vi "Create IO Channels.vi"(6 "AI Buffer Size (s)":i32=10, 8 "AI Block Size":i32=5000, 9 "OSC Configuration":T3(array[cluster])=[[{"Signal Type"=enum."Sine Wave", "DC"=0.0, "Amplitude"=0.01, "frequency"=2.0, "Phase"=0.0}, {"Signal Type"=enum."Sine Wave", "DC"=0.001, "Amplitude"=0.005, "frequency"=2.0, "Phase"=0.0}]] {"frequency" step=0.001 format="%.3p"; "Amplitude" format="%0.2p"; "DC" min=-0.99 max=0.99 format="%.2p"}, 10 "AO Configuration":T1(array[cluster])=[{"Output physical channels"="PXI1Slot2/ao0", "AO. Max"=0.1, "AO.Min"=-0.1}, {"Output physical channels"="", "AO. Max"=0.1, "AO.Min"=-0.1}], 11 "AI Configuration":T2(array[cluster])=[{"AI.Coupling"=10050, "AI.Max"=10.0, "AI.Min"=-10.0, "Input physical channels"="PXI1Slot2/ai0:1"}, {"AI.Coupling"=10050, "AI.Max"=10.0, "AI.Min"=-10.0, "Input physical channels"="PXI1Slot3/ai0:3"}, {"AI.Coupling"=10050, "AI.Max"=10.0, "AI.Min"=-10.0, "Input physical channels"=""}] {"AI.Coupling" items=["AC"=10045, "DC"=10050, "GND"=10066]}) -> (0 "Sampling information":cluster{"Fs":dbl, "#s":dbl}[](array[cluster])=[{"Fs"=10000.0, "#s"=5000.0}, {"Fs"=10000.0, "#s"=5000.0}], 1 "AI Rate":dbl=10000.0 format="%.2f", 2 "AO Task":refnum<k21>[](array[refnum]), 3 "AI task":refnum<k21>[](array[refnum]), 4 "phase log":dbl[](array[numeric])=[0.99999999999938, 0.99999999999938], 5 "appended array":errorcluster[][](array[cluster]))   [LabVIEW 2013]
uses:
  <vilib>/DAQmx/create/channels.llb/DAQmx Create Channel (AI-Voltage-Basic).vi
  <vilib>/DAQmx/configure/timing.llb/DAQmx Timing (Sample Clock).vi
  Lock-in Globals Multiple Inputs and Outputs.vi
  <vilib>/DAQmx/create/channels.llb/DAQmx Create Channel (AO-Voltage-Basic).vi
  <vilib>/DAQmx/configure/trigger.llb/DAQmx Start Trigger (Digital Edge).vi
  <vilib>/DAQmx/write.llb/DAQmx Write (Analog 1D Wfm NChan NSamp).vi
  <resource>/objmgr/daqmx.rc
  <vilib>/measure/NI_MABase.lvlib
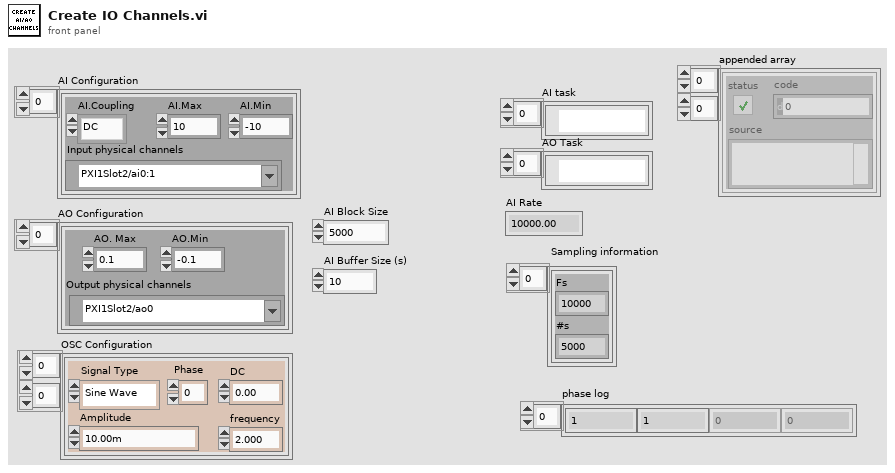
[diagram p1: front panel]
types:
  T1 = cluster{"Output physical channels":tag, "AO. Max":dbl, "AO.Min":dbl}[]
  T2 = cluster{"AI.Coupling":i32, "AI.Max":dbl, "AI.Min":dbl, "Input physical channels":tag}[]
  T3 = cluster{"Signal Type":enum16{"Sine Wave", "Triangle Wave", "Square Wave", "Sawtooth Wave"}, "DC":dbl, "Amplitude":dbl, "frequency":dbl, "Phase":dbl}[][]
  T4 = cluster{"AI.Coupling":i32, "AI.Max":dbl, "AI.Min":dbl, "Input physical channels":tag}
  T5 = cluster{"Signal Type":enum16{"Sine Wave", "Triangle Wave", "Square Wave", "Sawtooth Wave"}, "DC":dbl, "Amplitude":dbl, "frequency":dbl, "Phase":dbl}
  T6 = enum16{"Sine Wave", "Triangle Wave", "Square Wave", "Sawtooth Wave"}
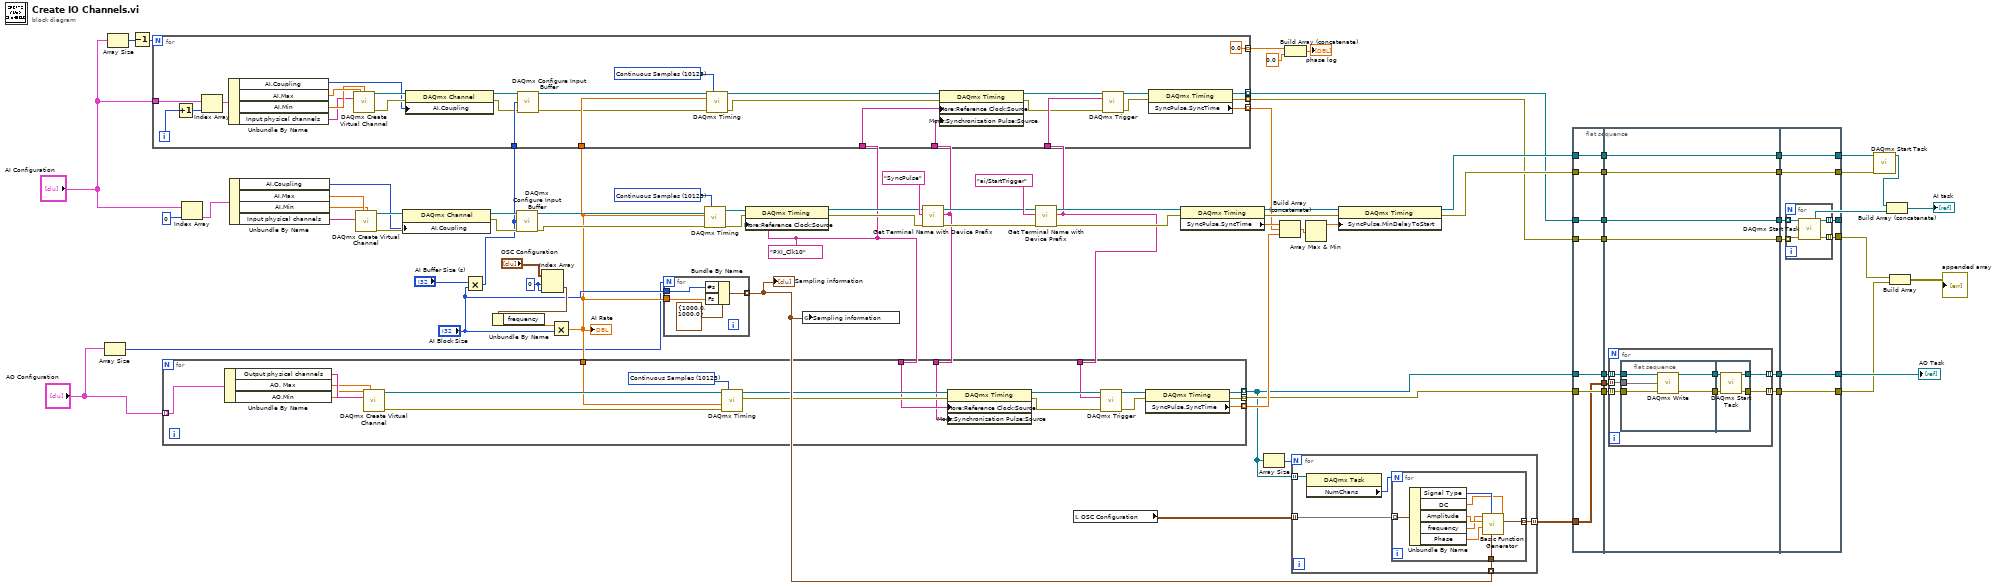
[diagram p0: block diagram]
diagram:
  w19 = 0 ("index (row)")
  w17 = tag "PXI_Clk10" ("RefClk.Src")
  w66 = 10123 items=["Finite Samples"=10178, "Continuous Samples"=10123] ("sample mode")
  n1 = Array Size(array="AO Configuration") -> (size(s)=w1:i32)
  n2 = Array Size(array="AI Configuration") -> (size(s)=w22:i32)
  n3 = Decrement(x=w22) -> (x-1=w21:i32)
  n4 = Index Array(array="AI Configuration", index=0) -> (element=w67:T4)
  n5 = Unbundle By Name(w67) -> ("AI.Coupling"=w39:i32, "AI.Max"=w46:dbl, "AI.Min"=w45:dbl, "Input physical channels"=w47:tag)
  n6 = call-poly <vilib>:"DAQmx Create Virtual Channel.vi"("maximum value"=w46, "minimum value"=w45, "physical channels"=w47) -> ("task out"=w41:refnum<k21>, "error out"=w40:errorcluster)  [unwired: 11 in]
  n7 = property class="DAQmx Channel"(reference=w41, error in=w40, "AI.Coupling"=w39) -> (reference out=w38:refnum<k21>, error out=w37:errorcluster)
  n8 = Multiply(x="AI Buffer Size (s)", y="AI Block Size") -> (x*y=w20:i32)
  n9 = call <vilib>:"DAQmx Configure Input Buffer.vi"("task/channels in"=w38, "buffer size (in samples per channel)"=w20, "error in"=w37) -> ("task out"=w36:refnum<k21>, "error out"=w35:errorcluster)  [unwired: 11 in]
  n10 = Index Array(array="OSC Configuration", index (row)=w19, index (col)=w19) -> (element=w30:T5)
  n11 = Unbundle By Name(w30) -> ("frequency"=w29:dbl)
  n12 = Multiply(x=w29, y="AI Block Size") -> (x*y=w18:dbl)
  "AI Rate" <- w18
  n13 = for {
    N: w1 -> [_]
    tunnel: w18 -> [w85]
    tunnel: "AI Block Size" -> [w84]
    tunnel: [w82] -> w8 mode=indexing
    n14 = Bundle By Name(cluster=cluster{"Fs":dbl, "#s":dbl} {"Fs"=1000.0, "#s"=1000.0} ("sampling info"), "#s"=w84, "Fs"=w85) -> (w82:cluster{"Fs":dbl, "#s":dbl})
  }
  "Sampling information" <- w8
  n15 = call-poly <vilib>:"DAQmx Timing.vi"("task/channels in"=w36, "sample mode"=w66, "rate"=w18, "error in"=w35) -> ("task out"=w65:refnum<k21>, "error out"=w64:errorcluster)  [unwired: 10 in]
  n16 = property class="DAQmx Timing"(reference=w65, error in=w64, "More:Reference Clock:Source"=w17) -> (reference out=w43:refnum<k21>, error out=w42:errorcluster)
  n17 = global write "Lock-in Globals Multiple Inputs and Outputs.vi" "Sampling information"(w8) -> ()
  n18 = call <userlib>:"Get Terminal Name with Device Prefix.vi"("error in (no error)"=w42, "Local Terminal Name"="SyncPulse", "task/channels in"=w43) -> ("error out"=w59:errorcluster, "Terminal Name with Device Prefix"=w16:tag, "task out"=w60:refnum<k21>)  [unwired: 6 in]
  n19 = call <userlib>:"Get Terminal Name with Device Prefix.vi"("error in (no error)"=w59, "Local Terminal Name"="ai/StartTrigger", "task/channels in"=w60) -> ("error out"=w57:errorcluster, "Terminal Name with Device Prefix"=w26:tag, "task out"=w58:refnum<k21>)  [unwired: 6 in]
  n20 = for {
    N: w21 -> [_]
    tunnel: "AI Configuration" -> [w113]
    tunnel: w20 -> [w115]
    tunnel: w18 -> [w114]
    tunnel: w17 -> [w112]
    tunnel: w16 -> [w111]
    tunnel: w26 -> [w110]
    tunnel: [w109] -> w25 mode=indexing
    tunnel: [w108] -> w23 mode=indexing
    tunnel: [w107] -> w24 mode=indexing
    tunnel: [0.0] -> w12 mode=indexing
    i -> [w88]
    w97 = 10123 items=["Finite Samples"=10178, "Continuous Samples"=10123, "Hardware Timed Single Point"=12522] ("sample mode")
    n21 = Increment(x=w88) -> (x+1=w87:i32)
    n22 = Index Array(array=w113, index=w87) -> (element=w96:T4)
    n23 = Unbundle By Name(w96) -> ("AI.Coupling"=w101:i32, "AI.Max"=w106:dbl, "AI.Min"=w105:dbl, "Input physical channels"=w104:tag)
    n24 = call-poly <vilib>:"DAQmx Create Virtual Channel.vi"("maximum value"=w106, "minimum value"=w105, "physical channels"=w104) -> ("task out"=w102:refnum<k21>, "error out"=w103:errorcluster)  [unwired: 11 in]
    n25 = property class="DAQmx Channel"(reference=w102, error in=w103, "AI.Coupling"=w101) -> (reference out=w100:refnum<k21>, error out=w99:errorcluster)
    n26 = call <vilib>:"DAQmx Configure Input Buffer.vi"("task/channels in"=w100, "buffer size (in samples per channel)"=w115, "error in"=w99) -> ("task out"=w98:refnum<k21>, "error out"=w91:errorcluster)  [unwired: 11 in]
    n27 = call-poly <vilib>:"DAQmx Timing.vi"("task/channels in"=w98, "sample mode"=w97, "rate"=w114, "error in"=w91) -> ("task out"=w95:refnum<k21>, "error out"=w90:errorcluster)  [unwired: 10 in]
    n28 = property class="DAQmx Timing"(reference=w95, error in=w90, "More:Reference Clock:Source"=w112, "More:Synchronization Pulse:Source"=w111) -> (reference out=w94:refnum<k21>, error out=w89:errorcluster)
    n29 = call-poly <vilib>:"DAQmx Trigger.vi"("task/channels in"=w94, "source"=w110, "error in"=w89) -> ("task out"=w93:refnum<k21>, "error out"=w92:errorcluster)  [unwired: 11 in]
    n30 = property class="DAQmx Timing"(reference=w93, error in=w92) -> (reference out=w107:refnum<k21>, error out=w108:errorcluster, "SyncPulse.SyncTime"=w109:dbl)
  }
  n31 = for {
    tunnel: [w128] -> w51 mode=indexing
    tunnel: [w127] -> w48 mode=indexing
    tunnel: [w121] -> w9 mode=indexing
    tunnel: w26 -> [w120]
    tunnel: "AO Configuration" -> [w116] mode=indexing
    tunnel: w18 -> [w119]
    tunnel: w17 -> [w118]
    tunnel: w16 -> [w117]
    w135 = 10123 items=["Finite Samples"=10178, "Continuous Samples"=10123] ("sample mode")
    n32 = Unbundle By Name(w116) -> ("Output physical channels"=w124:tag, "AO. Max"=w123:dbl, "AO.Min"=w122:dbl)
    n33 = call-poly <vilib>:"DAQmx Create Virtual Channel.vi"("maximum value"=w123, "minimum value"=w122, "physical channels"=w124) -> ("task out"=w126:refnum<k21>, "error out"=w125:errorcluster)  [unwired: 11 in]
    n34 = call-poly <vilib>:"DAQmx Timing.vi"("task/channels in"=w126, "sample mode"=w135, "rate"=w119, "error in"=w125) -> ("task out"=w134:refnum<k21>, "error out"=w133:errorcluster)  [unwired: 10 in]
    n35 = property class="DAQmx Timing"(reference=w134, error in=w133, "More:Reference Clock:Source"=w118, "More:Synchronization Pulse:Source"=w117) -> (reference out=w132:refnum<k21>, error out=w131:errorcluster)
    n36 = call-poly <vilib>:"DAQmx Trigger.vi"("task/channels in"=w132, "source"=w120, "error in"=w131) -> ("task out"=w129:refnum<k21>, "error out"=w130:errorcluster)  [unwired: 11 in]
    n37 = property class="DAQmx Timing"(reference=w129, error in=w130) -> (reference out=w121:refnum<k21>, error out=w127:errorcluster, "SyncPulse.SyncTime"=w128:dbl)
  }
  n38 = local read "OSC Configuration"() -> (w27:T3)
  n39 = property class="DAQmx Timing"(reference=w58, error in=w57) -> (reference out=w54:refnum<k21>, error out=w55:errorcluster, "SyncPulse.SyncTime"=w56:dbl)
  n40 = Array Size(array=w9) -> (size(s)=w10:i32)
  n41 = Build Array (concatenate)(w56, w25, w51) -> (w53:dbl[])
  n42 = Build Array (concatenate)(w12, 0.0) -> (→"phase log":dbl[])
  n43 = for {
    N: w10 -> [_]
    tunnel: w27 -> [w140] mode=indexing
    tunnel: [w139] -> w15 mode=indexing
    tunnel: w9 -> [w137] mode=indexing
    tunnel: w8 -> [w136] mode=indexing
    n44 = property class="DAQmx Task"(reference=w137) -> ("NumChans"=w138:u32)  [unwired: 1 in, 2 out]
    n45 = for {
      N: w138 -> [_]
      tunnel: w140 -> [w142] mode=indexing
      tunnel: [w143] -> w139 mode=indexing
      tunnel: w136 -> [w141]
      n46 = Unbundle By Name(w142) -> ("Signal Type"=w148:T6, "DC"=w147:dbl, "Amplitude"=w146:dbl, "frequency"=w145:dbl, "Phase"=w144:dbl)
      n47 = call <vilib>:"Basic Function Generator.vi"("offset"=w147, "sampling info"=w141, "signal type"=w148, "phase"=w144, "amplitude"=w146, "frequency"=w145) -> ("signal out"=w143:waveform(dbl))  [unwired: 3 in, 2 out]
    }
  }
  n48 = Array Max & Min(array=w53) -> (max value=w52:dbl)  [unwired: 3 out]
  n49 = property class="DAQmx Timing"(reference=w54, error in=w55, "SyncPulse.MinDelayToStart"=w52) -> (reference out=w49:refnum<k21>, error out=w50:errorcluster)
  n50 = flat-sequence {
    tunnel: w50 -> [w154]
    tunnel: w49 -> [w155]
    tunnel: [w155] -> w81
    tunnel: [w154] -> w80
    tunnel: [w153] -> w79
    tunnel: w48 -> [w153]
    tunnel: [w152] -> w78
    tunnel: w9 -> [w152]
    tunnel: [w149] -> w77
    tunnel: w15 -> [w149]
    tunnel: w24 -> [w151]
    tunnel: [w151] -> w76
    tunnel: [w150] -> w75
    tunnel: w23 -> [w150]
    tunnel: [w164] -> w74
    tunnel: [w163] -> w73
    tunnel: w81 -> [w164]
    tunnel: w80 -> [w163]
    tunnel: w79 -> [w162]
    tunnel: w78 -> [w161]
    tunnel: w77 -> [w160]
    tunnel: [w159] -> w72
    tunnel: w76 -> [w159]
    tunnel: [w158] -> w71
    tunnel: w75 -> [w158]
    tunnel: [w157] -> w70
    tunnel: [w156] -> w69
    tunnel: [w187] -> w5
    tunnel: [w188] -> w32
    tunnel: [w186] -> w63
    tunnel: [w185] -> w62
    tunnel: w74 -> [w186]
    tunnel: w73 -> [w185]
    tunnel: w72 -> [w184]
    tunnel: w71 -> [w183]
    tunnel: w70 -> [w181]
    tunnel: [w182] -> w14
    tunnel: w69 -> [w182]
    tunnel: [w181] -> w4
    frame #0 {
    }
    frame #1 {
      n51 = for {
        tunnel: w162 -> [w165] mode=indexing
        tunnel: w161 -> [w171] mode=indexing
        tunnel: w160 -> [w170] mode=indexing
        tunnel: [w167] -> w157 mode=indexing
        tunnel: [w166] -> w156 mode=indexing
        n52 = flat-sequence {
          tunnel: w165 -> [w176]
          tunnel: w171 -> [w175]
          tunnel: w170 -> [w172]
          tunnel: [w174] -> w169
          tunnel: [w173] -> w168
          tunnel: w169 -> [w180]
          tunnel: w168 -> [w177]
          tunnel: [w179] -> w167
          tunnel: [w178] -> w166
          frame #0 {
            n53 = call-poly <vilib>:"DAQmx Write.vi"("task/channels in"=w175, "data"=w172, "error in"=w176) -> ("task out"=w173:refnum<k21>, "error out"=w174:errorcluster)  [unwired: 10 in, 1 out]
          }
          frame #1 {
            n54 = call <vilib>:"DAQmx Start Task.vi"("task/channels in"=w177, "error in"=w180) -> ("task out"=w178:refnum<k21>, "error out"=w179:errorcluster)  [unwired: 12 in]
          }
        }
      }
    }
    frame #2 {
      n55 = for {
        tunnel: [w192] -> w188 mode=indexing
        tunnel: [w191] -> w187 mode=indexing
        tunnel: w184 -> [w190] mode=indexing
        tunnel: w183 -> [w189] mode=indexing
        n56 = call <vilib>:"DAQmx Start Task.vi"("task/channels in"=w190, "error in"=w189) -> ("task out"=w192:refnum<k21>, "error out"=w191:errorcluster)  [unwired: 12 in]
      }
    }
  }
  n57 = call <vilib>:"DAQmx Start Task.vi"("task/channels in"=w63, "error in"=w62) -> ("task out"=w33:refnum<k21>)  [unwired: 12 in, 1 out]
  n58 = Build Array (concatenate)(w33, w32) -> (→"AI task":refnum<k21>[])
  n59 = Build Array(w5, w4) -> (→"appended array":errorcluster[][])
  "AO Task" <- w14
